vi "Demo.vi"() -> ()   [LabVIEW 2011]
uses:
  Mirror Image(24 bit Vertical).vi
panel:
  out "Mirror Pic":picture
  out "Orin Pic":picture
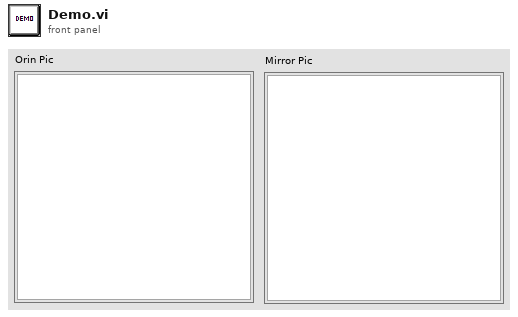
[diagram p1: front panel]
types:
  T1 = typedef "imagedata.ctl" = cluster{"image type":i32, "image depth":i32, "image":u8[], "mask":u8[], "colors":u32[], "Rectangle":cluster{"left":i16, "top":i16, "right":i16, "bottom":i16}}
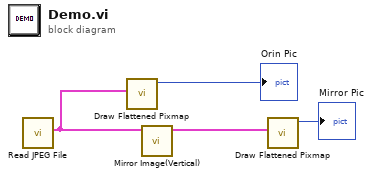
[diagram p0: block diagram]
diagram:
  n1 = call <vilib>:"Read JPEG File.vi"() -> ("image data"=w2:T1)  [unwired: 9 in, 2 out]
  n2 = call <vilib>:"Draw Flattened Pixmap.vi"("image data"=w2) -> ("new picture"=→"Orin Pic":picture)  [unwired: 8 in]
  n3 = call-poly "Mirror Image(Vertical).vi"("image In"=w2) -> ("image out"=w1:T1)  [unwired: 9 in, 1 out]
  n4 = call <vilib>:"Draw Flattened Pixmap.vi"("image data"=w1) -> ("new picture"=→"Mirror Pic":picture)  [unwired: 8 in]
